vi "Popup Menu Get State.vi"(11 "Error In":errorcluster) -> (8 "FP State":T1(ring), 15 "Error Out":errorcluster)   [LabVIEW 2020]
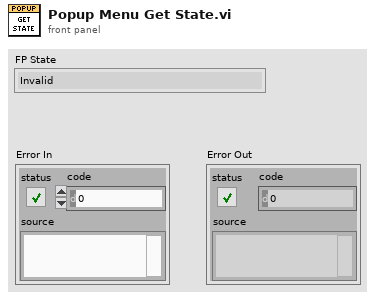
[diagram p1: front panel]
types:
  T1 = enum32{"Invalid", "Standard", "Closed", "Hidden", "Minimized", "Maximized"}
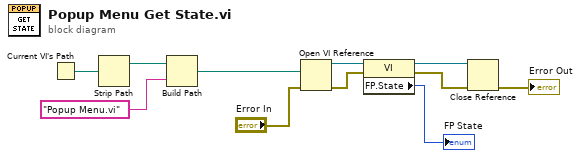
[diagram p0: block diagram]
diagram:
  n1 = Current VI's Path() -> (path=w4:path)
  n2 = Strip Path(path=w4) -> (stripped path=w3:path)  [unwired: 1 out]
  n3 = Build Path(base path=w3, name or relative path="Popup Menu.vi") -> (appended path=w1:path)
  n4 = Open VI Reference(vi path=w1, error in (no error)="Error In") -> (vi reference=w11:refnum<vi>, error out=w10:errorcluster)  [unwired: 4 in]
  n5 = property class="VI"(reference=w11, error in=w10) -> (reference out=w7:refnum<vi>, error out=w6:errorcluster, "FP.State"=→"FP State":T1)
  n6 = Close Reference(reference=w7, error in (no error)=w6) -> (error out=→"Error Out":errorcluster)
